vi "Read.vi"(7 "length":u16, 8 "error in (no error)":errorcluster, 9 "Start address":string, 10 "Read Type":variant, 11 "MelsecTCP in":refnum<class "InovanceSerial.lvclass">) -> (0 "error out":errorcluster, 2 "Data":variant, 3 "MelsecTCP out":refnum<class "InovanceSerial.lvclass">)   [LabVIEW 2020, in "HslCommunication.lvlib" / "InovanceSerial.lvclass"]
uses:
  InovanceSerial.lvclass
  D:/Git/Labview-Libraries/Libraries/HslCommunication/Abstract PLC Controler/Abstract PLC Controler.lvclass
  EventLogger.lvlibp/1abvi3w/vi.lib/gpm_packages/@cs/event-logger/Source/Composed Log/Types/Log Level.ctl
  Abstract PLC Controler/Abstract PLC Controler.lvclass/Abstract PLC Controler.ctl
  D:/Git/Labview-Libraries/Libraries/HslCommunication/_Dependenciecs/HslCommunication.dll
  _Dependenciecs/HslCommunication.dll
  Read reference.vi
  Abstract PLC Controler/Abstract PLC Controler.lvclass
  InovanceSerial.lvclass/InovanceSerial.ctl
  <vilib>/Utility/Data Type/NI_Data Type.lvlib
  EventLogger.lvlibp/Logger.lvclass
  EventLogger.lvlibp/1abvi3w/vi.lib/gpm_packages/@cs/event-logger/Source/Composed Log/Composed Log.lvlib
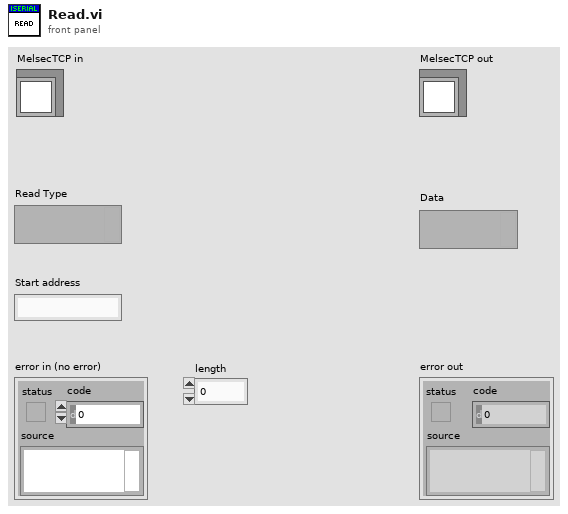
[diagram p1: front panel]
types:
  T1 = typedef "EventLogger.lvlibp/Composed Log.lvlib/Log Level.ctl" = enum16{"Debug", "Info", "Warning", "Error", "Critical"}
  T2 = typedef "NI_Data Type.lvlib/Data Type.ctl" = enum8{"Invalid Type", "Void", "I8", "I16", "I32", "I64", "U8", "U16", "U32", "U64", "Single Float", "Double Float", "Extended Float", "Single Complex", "Double Complex", "Extended Complex", "Enum U8", "Enum U16", "Enum U32", "Enum U64", "Single Float With Unit", "Double Float With Unit", "Extended Float With Unit", "Single Complex with Unit", "Double Complex with Unit", "Extended Complex with Unit", "Boolean", "String", "Path", "Picture", "Tag", "Array", "Cluster", "Variant", "LV Variant", "Waveform", "Timestamp", "Digital Waveform", "Digital Data", "ExpressData", "Refnum", "External Data", "VI", "Poly VI", "LabVIEW Class Instance", "Fixed Point", "Set Collection", "Map Collection"}
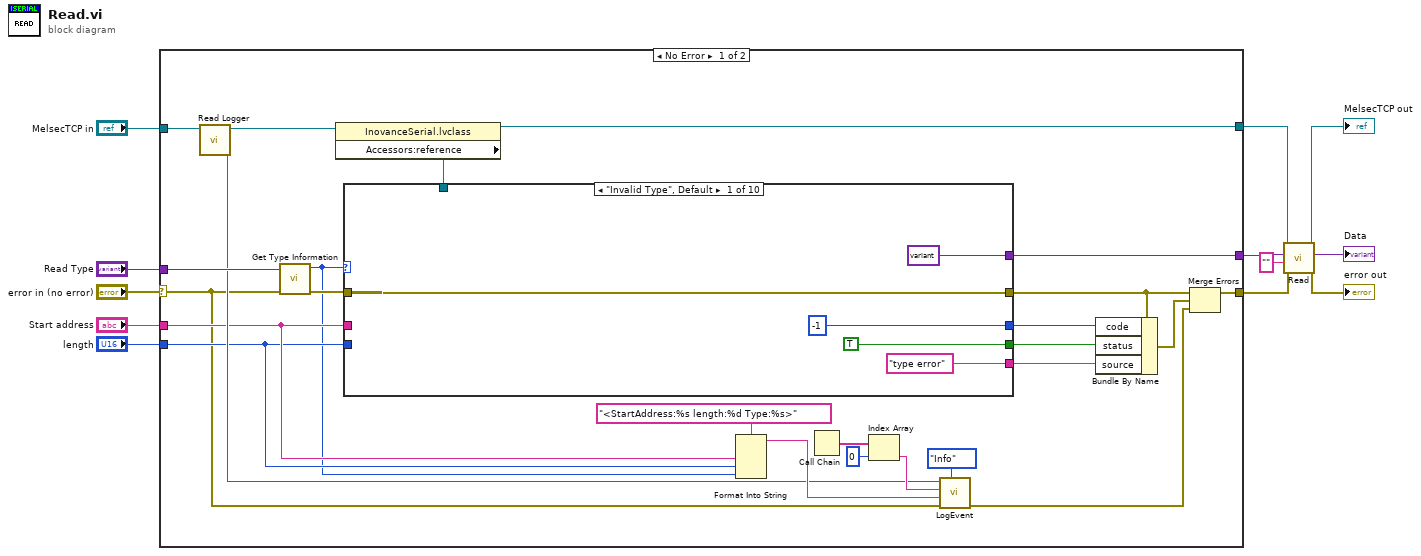
[diagram p0: block diagram]
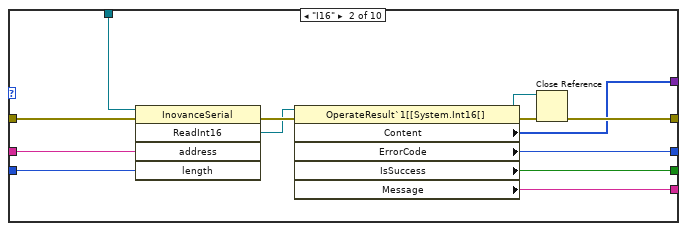
[diagram p2: hidden frame]
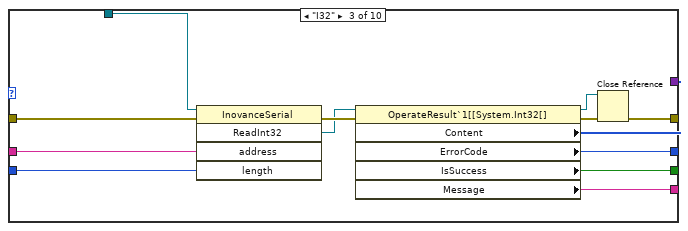
[diagram p3: hidden frame]
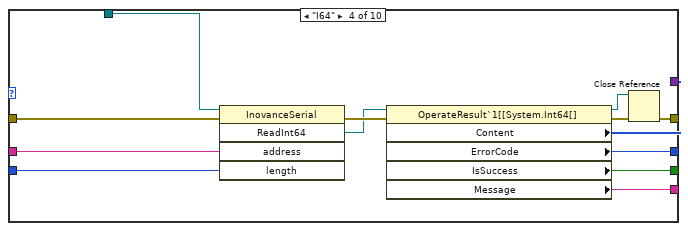
[diagram p4: hidden frame]
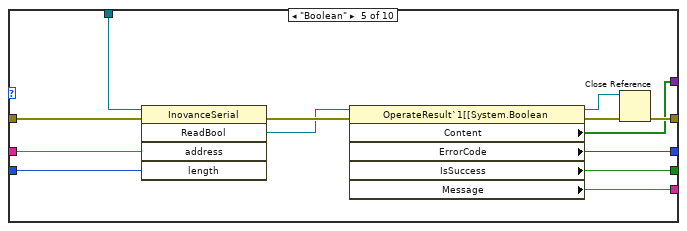
[diagram p5: hidden frame]
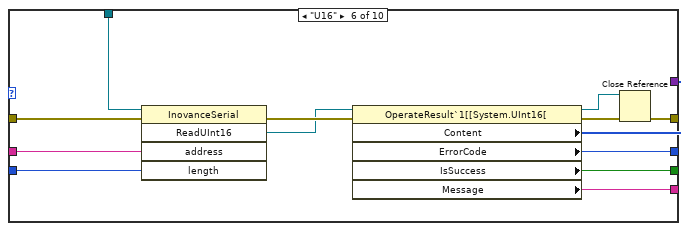
[diagram p6: hidden frame]
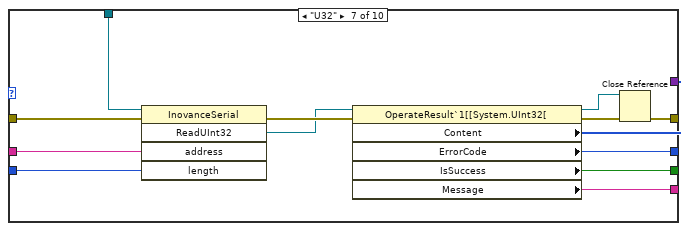
[diagram p7: hidden frame]
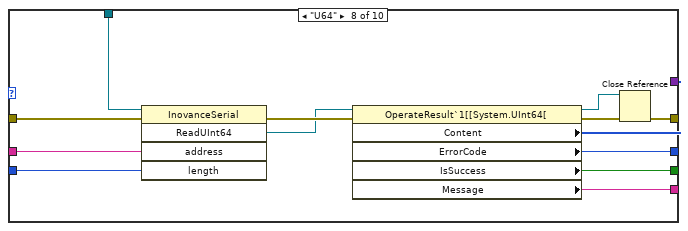
[diagram p8: hidden frame]
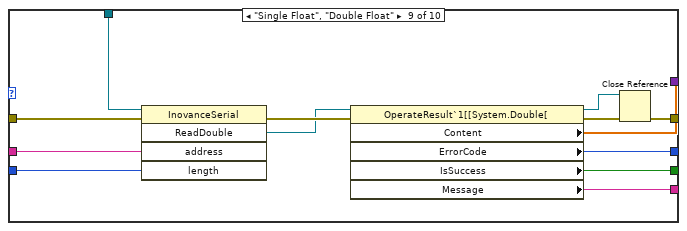
[diagram p9: hidden frame]
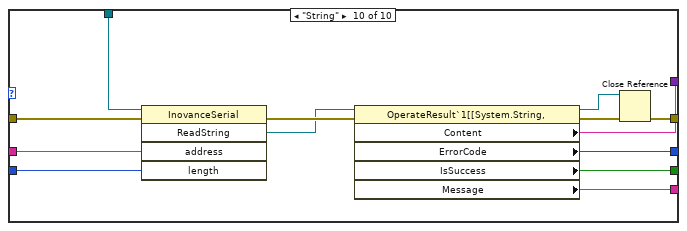
[diagram p10: hidden frame]
diagram:
  n1 = case shown="No Error" "error in (no error)" {
    selector: "error in (no error)" -> [w13 w162]
    tunnel: "MelsecTCP in" -> [w37 w161]
    tunnel: [w28 w161] -> w5
    tunnel: "Start address" -> [w16 _]
    tunnel: [w34 w162] -> w8
    tunnel: [w35 w160] -> w3
    tunnel: "length" -> [w15 _]
    tunnel: "Read Type" -> [w27 w160]
    frame No Error {
      n2 = call "Read Logger.vi"("Abstract PLC Controler in"=w37) -> ("EventLogger.lvlibp:Logger.lvclass"=w18:refnum<class "Logger.lvclass">, "Abstract PLC Controler out"=w19:refnum<class "InovanceSerial.lvclass">)  [unwired: 9 in]
      n3 = call <vilib>:"Get Type Information.vi"("error in (no error)"=w13, "variant"=w27) -> ("error out"=w26:errorcluster, "type"=w14:T2)  [unwired: 5 in, 3 out]
      n4 = property class="InovanceSerial.lvclass"(reference=w19) -> (reference out=w28:refnum<class "InovanceSerial.lvclass">, "Accessors:reference"=w36:refnum<k24>)  [unwired: 1 in, 1 out]
      n5 = case shown="\"Invalid Type\", Default" w14 {
        tunnel: w36 -> [_ w55 w68 w81 w83 w96 w109 w122 w135 w148]
        tunnel: w16 -> [_ w54 w67 w80 w94 w107 w120 w133 w146 w159]
        tunnel: w15 -> [_ w53 w66 w79 w93 w106 w119 w132 w145 w158]
        tunnel: w26 -> [w42 w52 w65 w78 w92 w105 w118 w131 w144 w157]
        tunnel: [w42 w47 w60 w73 w87 w100 w113 w126 w139 w152] -> w30
        tunnel: [variant ("Read Type") w43 w56 w69 w82 w95 w108 w121 w134 w147] -> w35
        tunnel: [-1 ("ErrorCode") w46 w59 w72 w86 w99 w112 w125 w138 w151] -> w33
        tunnel: [TRUE ("IsSuccess") w45 w58 w71 w85 w98 w111 w124 w137 w150] -> w32
        tunnel: ["type error" ("Message") w44 w57 w70 w84 w97 w110 w123 w136 w149] -> w31
        frame "Invalid Type", Default {
        }
        frame "I16" {
          n6 = invoke class="InovanceSerial" method="ReadInt16"(reference=w55, error in=w52, "address"=w54, "length"=w53) -> (error out=w51:errorcluster, "ReadInt16"=w49:refnum<k24>)  [unwired: 1 in, 3 out]
          n7 = property class="OperateResult`1[[System.Int16[]"(reference=w49, error in=w51) -> (reference out=w48:refnum<k24>, error out=w50:errorcluster, "Content"=w43:i16[], "ErrorCode"=w46:i32, "IsSuccess"=w45:bool, "Message"=w44:string)
          n8 = Close Reference(reference=w48, error in (no error)=w50) -> (error out=w47:errorcluster)
        }
        frame "I32" {
          n9 = invoke class="InovanceSerial" method="ReadInt32"(reference=w68, error in=w65, "address"=w67, "length"=w66) -> (error out=w64:errorcluster, "ReadInt32"=w62:refnum<k24>)  [unwired: 1 in, 3 out]
          n10 = property class="OperateResult`1[[System.Int32[]"(reference=w62, error in=w64) -> (reference out=w61:refnum<k24>, error out=w63:errorcluster, "Content"=w56:i32[], "ErrorCode"=w59:i32, "IsSuccess"=w58:bool, "Message"=w57:string)
          n11 = Close Reference(reference=w61, error in (no error)=w63) -> (error out=w60:errorcluster)
        }
        frame "I64" {
          n12 = invoke class="InovanceSerial" method="ReadInt64"(reference=w81, error in=w78, "address"=w80, "length"=w79) -> (error out=w77:errorcluster, "ReadInt64"=w75:refnum<k24>)  [unwired: 1 in, 3 out]
          n13 = property class="OperateResult`1[[System.Int64[]"(reference=w75, error in=w77) -> (reference out=w74:refnum<k24>, error out=w76:errorcluster, "Content"=w69:i64[], "ErrorCode"=w72:i32, "IsSuccess"=w71:bool, "Message"=w70:string)
          n14 = Close Reference(reference=w74, error in (no error)=w76) -> (error out=w73:errorcluster)
        }
        frame "Boolean" {
          n15 = invoke class="InovanceSerial" method="ReadBool"(reference=w83, error in=w92, "address"=w94, "length"=w93) -> (error out=w91:errorcluster, "ReadBool"=w89:refnum<k24>)  [unwired: 1 in, 3 out]
          n16 = property class="OperateResult`1[[System.Boolean"(reference=w89, error in=w91) -> (reference out=w88:refnum<k24>, error out=w90:errorcluster, "Content"=w82:bool[], "ErrorCode"=w86:i32, "IsSuccess"=w85:bool, "Message"=w84:string)
          n17 = Close Reference(reference=w88, error in (no error)=w90) -> (error out=w87:errorcluster)
        }
        frame "U16" {
          n18 = invoke class="InovanceSerial" method="ReadUInt16"(reference=w96, error in=w105, "address"=w107, "length"=w106) -> (error out=w104:errorcluster, "ReadUInt16"=w102:refnum<k24>)  [unwired: 1 in, 3 out]
          n19 = property class="OperateResult`1[[System.UInt16["(reference=w102, error in=w104) -> (reference out=w101:refnum<k24>, error out=w103:errorcluster, "Content"=w95:u16[], "ErrorCode"=w99:i32, "IsSuccess"=w98:bool, "Message"=w97:string)
          n20 = Close Reference(reference=w101, error in (no error)=w103) -> (error out=w100:errorcluster)
        }
        frame "U32" {
          n21 = invoke class="InovanceSerial" method="ReadUInt32"(reference=w109, error in=w118, "address"=w120, "length"=w119) -> (error out=w117:errorcluster, "ReadUInt32"=w115:refnum<k24>)  [unwired: 1 in, 3 out]
          n22 = property class="OperateResult`1[[System.UInt32["(reference=w115, error in=w117) -> (reference out=w114:refnum<k24>, error out=w116:errorcluster, "Content"=w108:u32[], "ErrorCode"=w112:i32, "IsSuccess"=w111:bool, "Message"=w110:string)
          n23 = Close Reference(reference=w114, error in (no error)=w116) -> (error out=w113:errorcluster)
        }
        frame "U64" {
          n24 = invoke class="InovanceSerial" method="ReadUInt64"(reference=w122, error in=w131, "address"=w133, "length"=w132) -> (error out=w130:errorcluster, "ReadUInt64"=w128:refnum<k24>)  [unwired: 1 in, 3 out]
          n25 = property class="OperateResult`1[[System.UInt64["(reference=w128, error in=w130) -> (reference out=w127:refnum<k24>, error out=w129:errorcluster, "Content"=w121:u64[], "ErrorCode"=w125:i32, "IsSuccess"=w124:bool, "Message"=w123:string)
          n26 = Close Reference(reference=w127, error in (no error)=w129) -> (error out=w126:errorcluster)
        }
        frame "Single Float", "Double Float" {
          n27 = invoke class="InovanceSerial" method="ReadDouble"(reference=w135, error in=w144, "address"=w146, "length"=w145) -> (error out=w143:errorcluster, "ReadDouble"=w141:refnum<k24>)  [unwired: 1 in, 3 out]
          n28 = property class="OperateResult`1[[System.Double["(reference=w141, error in=w143) -> (reference out=w140:refnum<k24>, error out=w142:errorcluster, "Content"=w134:dbl[], "ErrorCode"=w138:i32, "IsSuccess"=w137:bool, "Message"=w136:string)
          n29 = Close Reference(reference=w140, error in (no error)=w142) -> (error out=w139:errorcluster)
        }
        frame "String" {
          n30 = invoke class="InovanceSerial" method="ReadString"(reference=w148, error in=w157, "address"=w159, "length"=w158) -> (error out=w156:errorcluster, "ReadString"=w154:refnum<k24>)  [unwired: 1 in, 3 out]
          n31 = property class="OperateResult`1[[System.String,"(reference=w154, error in=w156) -> (reference out=w153:refnum<k24>, error out=w155:errorcluster, "Content"=w147:string, "ErrorCode"=w151:i32, "IsSuccess"=w150:bool, "Message"=w149:string)
          n32 = Close Reference(reference=w153, error in (no error)=w155) -> (error out=w152:errorcluster)
        }
      }
      n33 = Format Into String(format string="<StartAddress:%s length:%d Type:%s>", w16, w15, w14) -> (resulting string=w22:string)  [unwired: 2 in, 1 out]
      n34 = Call Chain() -> (call chain=w25:string[])
      n35 = Index Array(array=w25, index=0) -> (element=w21:string)
      n36 = call "LogEvent.vi"("Event Level"=Log_Level."Info", "error in (no error)"=w13, "Data To Log"=w22, "SourceID"=w21, "Logger in"=w18) -> ("error out"=w17:errorcluster)  [unwired: 5 in, 1 out]
      n37 = Bundle By Name(cluster=w30, "code"=w33, "status"=w32, "source"=w31) -> (w29:errorcluster)
      n38 = Merge Errors(w30, w29, w17) -> (w34:errorcluster)
    }
    frame Error {
    }
  }
  n39 = call-parent "Read.vi"("error in (no error)"=w8, "Start address"="", "Read Type"=w3, "MelsecTCP in"=w5) -> ("error out"=→"error out":errorcluster, "Data"=→"Data":variant, "MelsecTCP out"=→"MelsecTCP out":refnum<class "InovanceSerial.lvclass">)  [unwired: 5 in]
